vi "background writer.vi"(0 "dictionary":T2, 1 "command queue":refnum<k33>, 2 "response from processor":refnum<k33>, 5 "logging path":path, 7 "backup directory":path, 9 "default data table":T1, 11 "scans per write":u16=20, 13 "enable channel (bool)":i32, 14 "has enable channel":bool) -> (15 "error out":errorcluster)   [LabVIEW 2013, in "Binary datalogger runtime.lvclass"]
uses:
  Binary datalogger runtime.lvclass
  <vilib>/NI/Tag Bus/dictionary/full data dictionary.ctl
  message to background process.ctl
  control enum.ctl
  <vilib>/NI/Tag Bus/table/data table.ctl
  response from background process.ctl
  response enum.ctl
  writer state enum.ctl
  data cache.ctl
  <vilib>/NI/Tag Bus/table/data table.lvlib
  <vilib>/NI/Configuration Framework/serializable configuration/NISE_CEF_serializable configuration.lvclass
  <vilib>/NI/Tag Bus/dictionary/data dictionary.lvclass
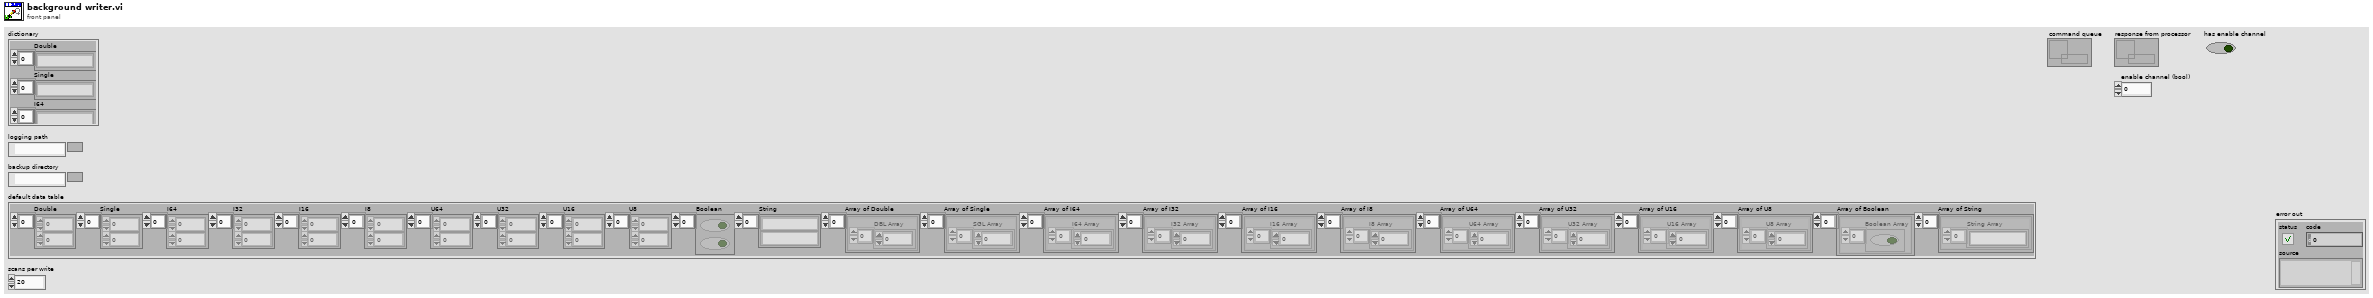
[diagram p1: front panel]
types:
  T1 = typedef "tag bus.lvlib/data table.lvlib/data table.ctl" = cluster{"Double":dbl[], "Single":sgl[], "I64":i64[], "I32":i32[], "I16":i16[], "I8":i8[], "U64":u64[], "U32":u32[], "U16":u16[], "U8":u8[], "Boolean":bool[], "String":string[], "Array of Double":cluster{"DBL Array":dbl[]}[], "Array of Single":cluster{"SGL Array":sgl[]}[], "Array of I64":cluster{"I64 Array":i64[]}[], "Array of I32":cluster{"I32 Array":i32[]}[], "Array of I16":cluster{"I16 Array":i16[]}[], "Array of I8":cluster{"I8 Array":i8[]}[], "Array of U64":cluster{"U64 Array":u64[]}[], "Array of U32":cluster{"U32 Array":u32[]}[], "Array of U16":cluster{"U16 Array":u16[]}[], "Array of U8":cluster{"U8 Array":u8[]}[], "Array of Boolean":cluster{"Boolean Array":bool[]}[], "Array of String":cluster{"String Array":string[]}[]}
  T2 = typedef "tag bus.lvlib/data dictionary.lvclass/full data dictionary.ctl" = cluster{"Double":string[], "Single":string[], "I64":string[], "I32":string[], "I16":string[], "I8":string[], "U64":string[], "U32":string[], "U16":string[], "U8":string[], "Boolean":string[], "String":string[], "Array of Double":string[], "Array of Single":string[], "Array of I64":string[], "Array of I32":string[], "Array of I16":string[], "Array of I8":string[], "Array of U64":string[], "Array of U32":string[], "Array of U16":string[], "Array of U8":string[], "Array of Boolean":string[], "Array of String":string[]}
  T3 = enum16{"open", "replace", "create", "open or create", "replace or create", "replace or create with confirmation"}
  T4 = typedef "Binary datalogger runtime.lvclass/data cache.ctl" = cluster{"timestamps":timestamp[], "dataset":T1[]}
  T5 = typedef "Binary datalogger runtime.lvclass/writer state enum.ctl" = enum16{"wait for message", "create file", "report error", "exit", "close file"}
  T6 = typedef "Binary datalogger runtime.lvclass/response enum.ctl" = enum16{"exit", "return buffer", "error"}
  T7 = typedef "Binary datalogger runtime.lvclass/response from background process.ctl" = cluster{"response enum":T6, "datapack":refnum<data-value>, "error code":i32}
  T8 = typedef "Binary datalogger runtime.lvclass/message to background process.ctl" = cluster{"control enum":T9, "datapack":refnum<data-value>, "Time Stamp":timestamp}
  T9 = typedef "Binary datalogger runtime.lvclass/control enum.ctl" = enum16{"exit", "output data"}
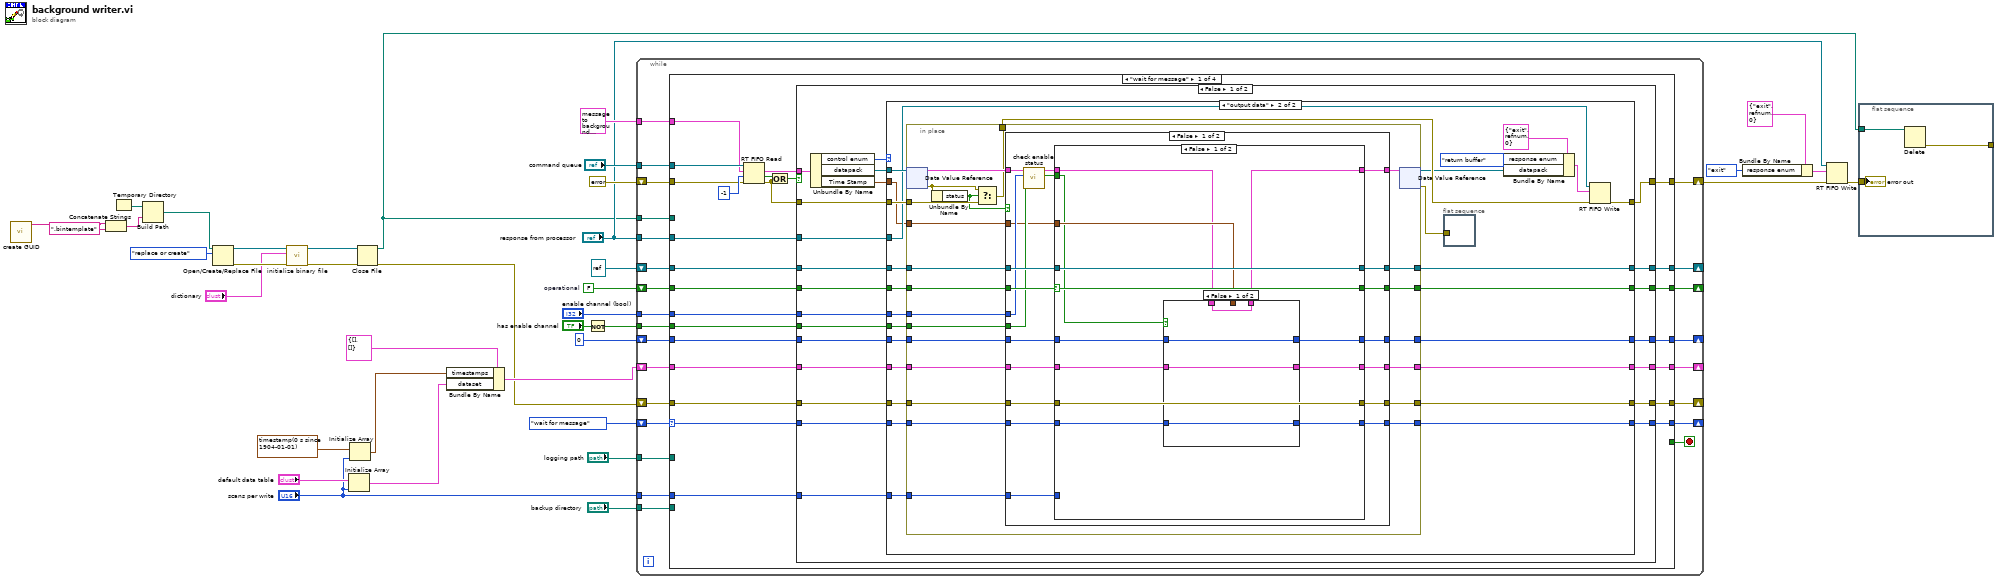
[diagram p0: block diagram]
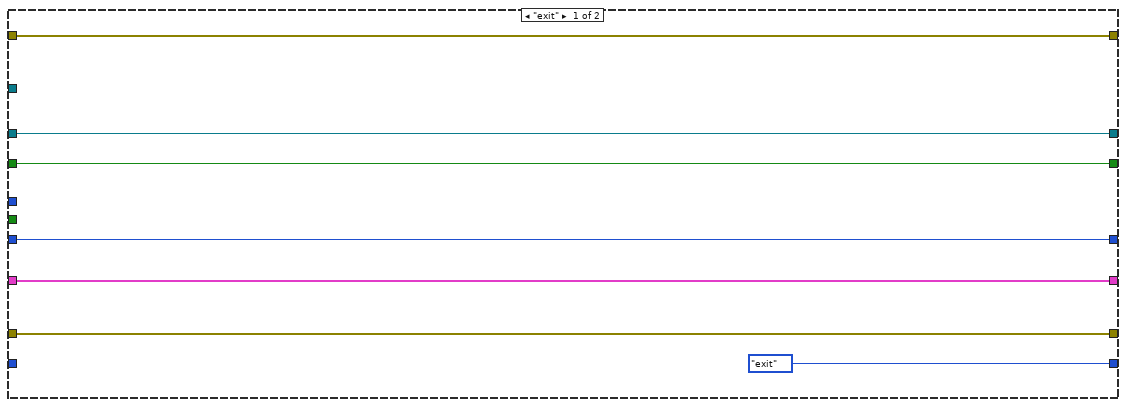
[diagram p2: hidden frame]
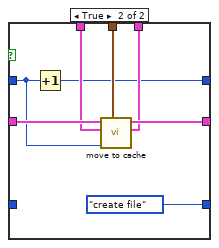
[diagram p3: hidden frame]
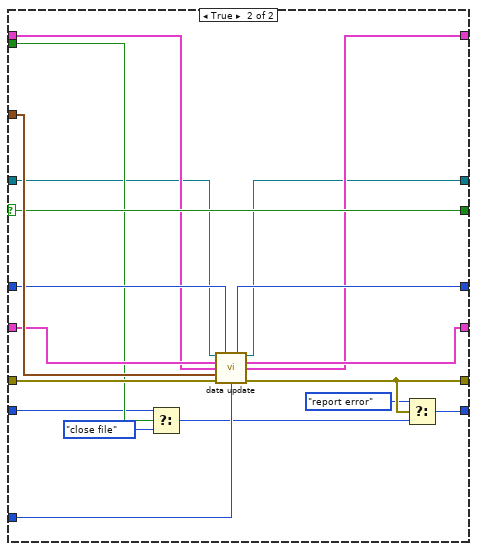
[diagram p4: hidden frame]
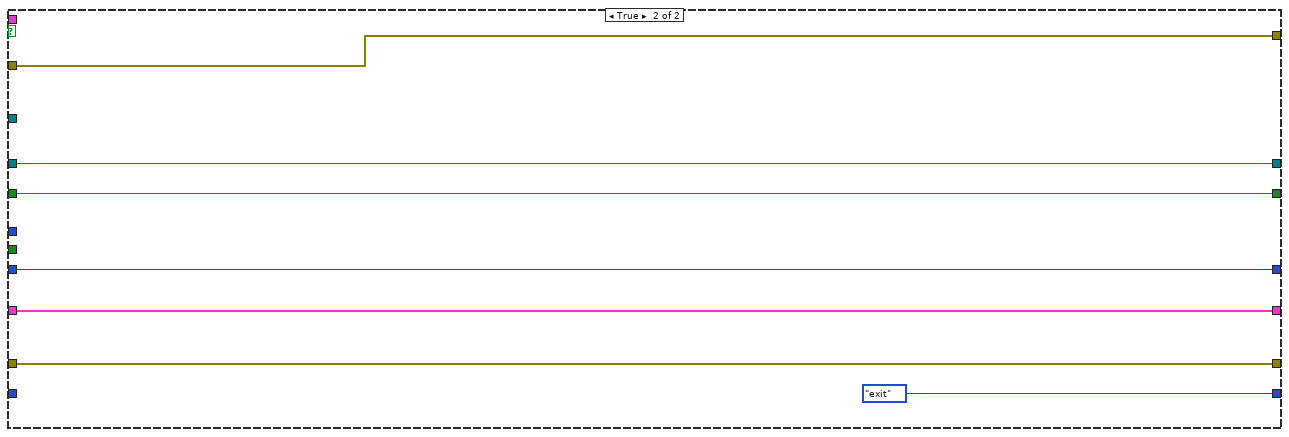
[diagram p6: hidden frame]
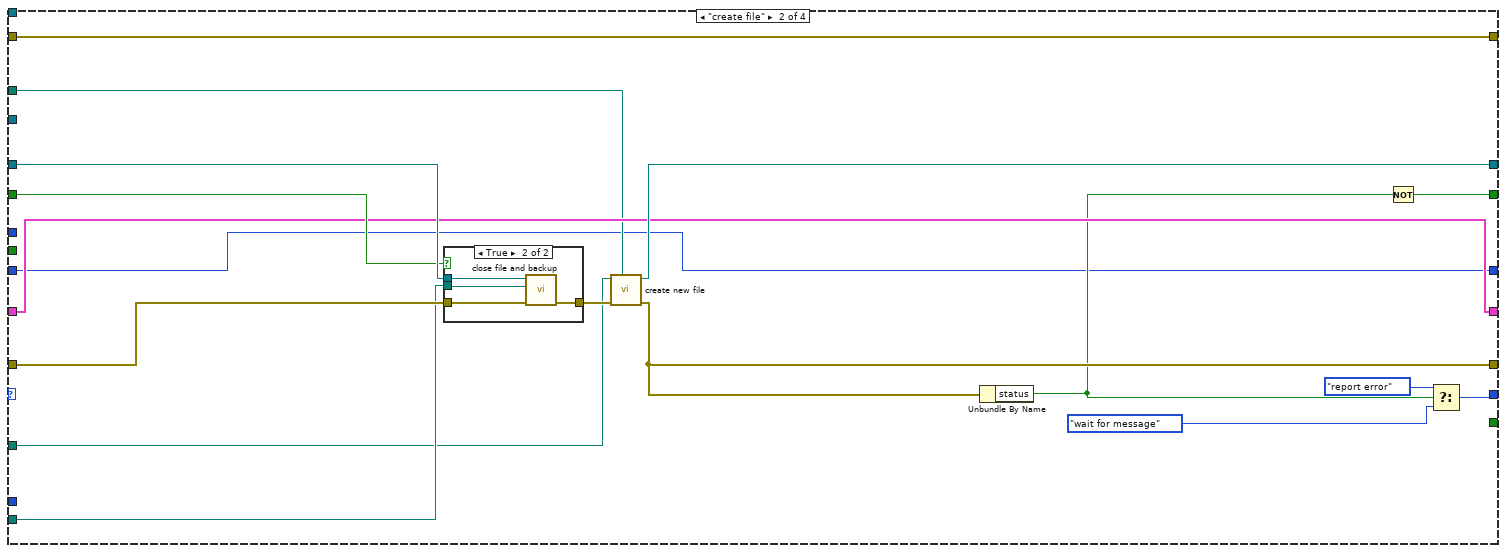
[diagram p7: hidden frame]
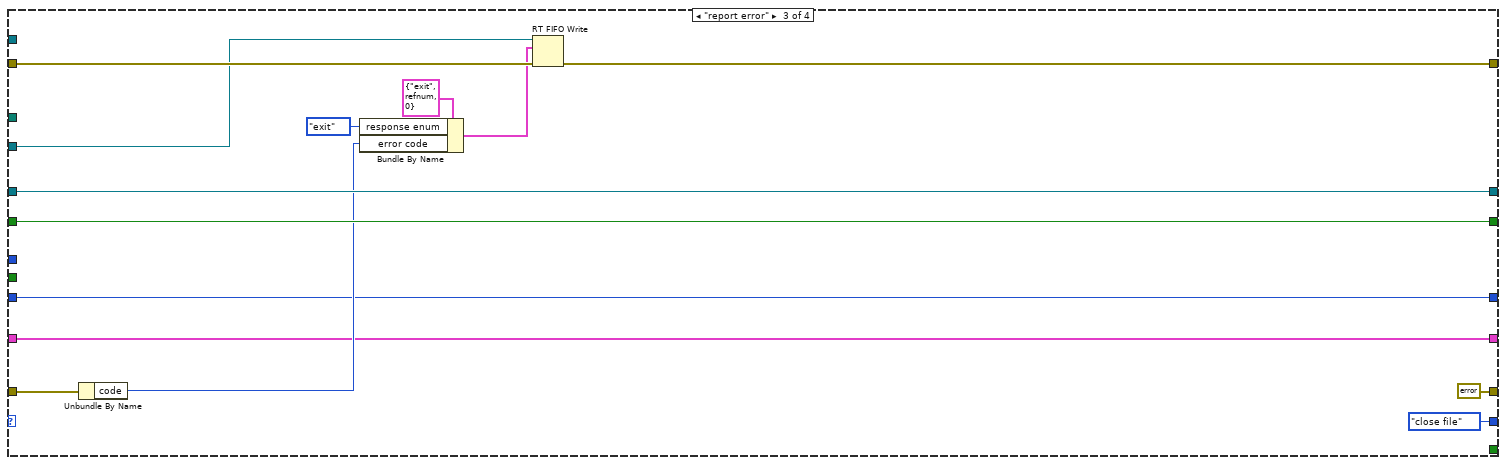
[diagram p9: hidden frame]
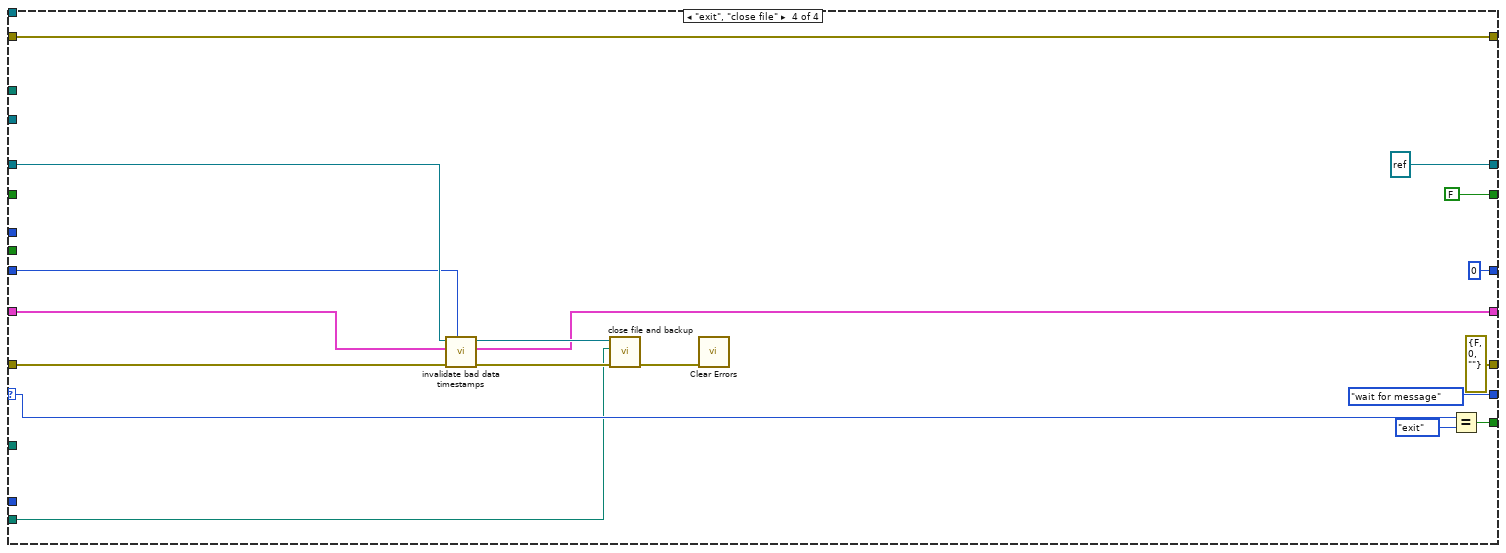
[diagram p10: hidden frame]
diagram:
  w28 = FALSE  # operational
  n1 = call <vilib>:"create GUID.vi"() -> ("uuid"=w12:string)  [unwired: 10 in, 1 out]
  n2 = Concatenate Strings(w12, ".bintemplate" ("string")) -> (w10:string)
  n3 = Temporary Directory() -> (w13:path)
  n4 = Build Path(base path=w13, name or relative path=w10) -> (appended path=w9:path)
  n5 = Open/Create/Replace File(file path (use dialog)=w9, operation (0:open)=T3."replace or create") -> (refnum out=w7:refnum<file>, error out=w6:errorcluster)  [unwired: 4 in, 1 out]
  n6 = call "initialize binary file.vi"("error in"=w6, "dictionary"="dictionary", "Byte Stream File in"=w7) -> ("error out"=w5:errorcluster, "Byte Stream File out"=w4:refnum<file>)  [unwired: 7 in]
  n7 = Initialize Array("default data table", "scans per write") -> (w17:T1[])
  n8 = Initialize Array(timestamp(0 s since 1904-01-01) ("Time Stamp"), "scans per write") -> (w14:timestamp[])
  n9 = Close File(refnum=w4, error in=w5) -> (path=w2:path, error out=w3:errorcluster)
  n10 = Bundle By Name(cluster=T4 {"timestamps"=[], "dataset"=[]} ("cache allocation in"), "timestamps"=w14, "dataset"=w17) -> (w18:T4)
  n11 = Not(x="has enable channel") -> (.not. x?=w24:bool)
  n12 = while {
    tunnel: "command queue" -> [w62]
    tunnel: T8 {"control enum"=enum."exit", "datapack"=refnum, "Time Stamp"=timestamp(0 s since 1904-01-01)} ("element") -> [w61]
    shift-right: [w59] -> w35
    shift-left: errorcluster {"status"=FALSE, "code"=0, "source"=""} ("error in") -> [w60]
    tunnel: "response from processor" -> [w57]
    shift-right: [w55] -> _
    shift-left: writer_state_enum."wait for message" ("logger state") -> [w56]
    shift-right: [w53] -> _
    shift-left: refnum<file> refnum ("refnum out") -> [w54]
    shift-right: [w46] -> _
    shift-left: w28 -> [w52]
    shift-right: [w50] -> _
    shift-left: w3 -> [w51]
    tunnel: "logging path" -> [w49]
    tunnel: "scans per write" -> [w48]
    tunnel: "backup directory" -> [w47]
    shift-right: [w45] -> _
    shift-left: 0 ("sample counter") -> [w44]
    shift-right: [w40] -> _
    shift-left: w18 -> [w41]
    tunnel: "enable channel (bool)" -> [w42]
    tunnel: w24 -> [w43]
    tunnel: w2 -> [w39]
    stop <- w58 stop-if-true
    n13 = case shown="\"wait for message\"" w56 {
      selector: w56 -> [w66 _ _ w294]
      tunnel: w62 -> [w87 _ _ _]
      tunnel: w61 -> [w85 _ _ _]
      tunnel: w60 -> [w84 w248 w278 w296]
      tunnel: [w80 w248 w276 w296] -> w59
      tunnel: [_ _ _ w295] -> w58
      tunnel: w57 -> [w78 _ w275 _]
      tunnel: [w77 w250 writer_state_enum."close file" ("logger state") writer_state_enum."wait for message" ("logger state")] -> w55
      tunnel: w54 -> [w76 w255 w277 w288]
      tunnel: [w75 w259 w277 refnum<file> refnum ("refnum out")] -> w53
      tunnel: w52 -> [w73 w247 w269 _]
      tunnel: w51 -> [w71 w256 w268 w289]
      tunnel: [w72 w258 errorcluster {"status"=FALSE, "code"=0, "source"=""} ("error out") errorcluster {"status"=FALSE, "code"=0, "source"=""} ("error out")] -> w50
      tunnel: w49 -> [_ w253 _ _]
      tunnel: w48 -> [w63 _ _ _]
      tunnel: w47 -> [_ w254 _ w287]
      tunnel: [w74 w249 w269 FALSE] -> w46
      tunnel: [w69 w243 w265 0 ("sample counter")] -> w45
      tunnel: w44 -> [w70 w243 w265 w284]
      tunnel: w43 -> [w64 _ _ _]
      tunnel: w42 -> [w65 _ _ _]
      tunnel: w41 -> [w68 w246 w266 w286]
      tunnel: [w67 w246 w266 w285] -> w40
      tunnel: w39 -> [_ w245 _ _]
      frame "wait for message" {
        n14 = RT FIFO Read(0:w87, 1:w85, 2:-1 ("timeout in ms (0)"), 3:w84) -> (9:w79:T8, 10:w83:bool, 11:w81:errorcluster)  [unwired: 2 out]
        n15 = Or(x=w83, y=w81) -> (x .or. y?=w82:bool)
        n16 = case shown="False" w82 {
          tunnel: w81 -> [w106 w242]
          tunnel: [w107 w242] -> w80
          tunnel: w79 -> [w109 _]
          tunnel: w78 -> [w103 _]
          tunnel: [w102 writer_state_enum."exit" ("logger state")] -> w77
          tunnel: w76 -> [w101 w240]
          tunnel: [w100 w240] -> w75
          tunnel: [w98 w239] -> w74
          tunnel: w73 -> [w99 w239]
          tunnel: [w97 w238] -> w72
          tunnel: w71 -> [w96 w238]
          tunnel: w70 -> [w94 w237]
          tunnel: [w95 w237] -> w69
          tunnel: w68 -> [w93 w236]
          tunnel: [w92 w236] -> w67
          tunnel: w66 -> [w91 _]
          tunnel: w65 -> [w90 _]
          tunnel: w64 -> [w89 _]
          tunnel: w63 -> [w88 _]
          frame False {
            n17 = Unbundle By Name(w109) -> ("control enum"=w108:T9, "datapack"=w104:refnum<data-value>, "Time Stamp"=w105:timestamp)
            n18 = case shown="\"output data\"" w108 {
              tunnel: [w116 w126] -> w107
              tunnel: w106 -> [w116 w141]
              tunnel: w105 -> [_ w118]
              tunnel: w104 -> [_ w142]
              tunnel: w103 -> [_ w123]
              tunnel: [writer_state_enum."exit" ("logger state") w130] -> w102
              tunnel: w101 -> [w114 w140]
              tunnel: [w114 w139] -> w100
              tunnel: w99 -> [w113 w137]
              tunnel: [w113 w138] -> w98
              tunnel: [w112 w131] -> w97
              tunnel: w96 -> [w112 w132]
              tunnel: [w110 w135] -> w95
              tunnel: w94 -> [w110 w136]
              tunnel: w93 -> [w111 w133]
              tunnel: [w111 w134] -> w92
              tunnel: w91 -> [_ w129]
              tunnel: w90 -> [_ w128]
              tunnel: w89 -> [_ w127]
              tunnel: w88 -> [_ w117]
              frame "exit" {
              }
              frame "output data" {
                n19 = in-place {
                  in-place-border: w141 -> [w164]
                  in-place-border: w140 -> [w159]
                  in-place-border: [w158] -> w139
                  in-place-border: [w157] -> w138
                  in-place-border: w137 -> [w156]
                  in-place-border: w136 -> [w155]
                  in-place-border: [w154] -> w135
                  in-place-border: [w153] -> w134
                  in-place-border: w133 -> [w152]
                  in-place-border: w132 -> [w151]
                  in-place-border: [w150] -> w131
                  in-place-border: [w149] -> w130
                  in-place-border: w129 -> [w148]
                  in-place-border: [w147] -> w125
                  in-place-border: w128 -> [w146]
                  in-place-border: w127 -> [w145]
                  in-place-border: w118 -> [w144]
                  in-place-border: w117 -> [w143]
                  n20 = in-place-dvr #1(w142) -> (w160:T1, w163:errorcluster)
                  n21 = Unbundle By Name(w163) -> ("status"=w162:bool)
                  n22 = Select(t=w163, s=w162, f=w164) -> (s? t:f=w147:errorcluster)
                  n23 = case shown="False" w162 {
                    tunnel: [w169 w235] -> w161
                    tunnel: w160 -> [w172 w235]
                    tunnel: w159 -> [w181 w234]
                    tunnel: [w182 w234] -> w158
                    tunnel: [w183 w233] -> w157
                    tunnel: w156 -> [w184 w233]
                    tunnel: w155 -> [w179 w232]
                    tunnel: [w180 w232] -> w154
                    tunnel: [w175 w231] -> w153
                    tunnel: w152 -> [w176 w231]
                    tunnel: w151 -> [w178 w230]
                    tunnel: [w177 w230] -> w150
                    tunnel: [w174 w229] -> w149
                    tunnel: w148 -> [w173 w229]
                    tunnel: w146 -> [w168 _]
                    tunnel: w145 -> [w167 _]
                    tunnel: w144 -> [w166 _]
                    tunnel: w143 -> [w165 _]
                    frame False {
                      n24 = call "check enable status.vi"("always enabled?"=w167, "enable channel index"=w168, "data table in"=w172) -> ("enabled?"=w170:bool, "Data table out"=w171:T1)  [unwired: 7 in]
                      n25 = case shown="False" w184 {
                        selector: w184 -> [w197 w222]
                        tunnel: [w197 w222] -> w183
                        tunnel: [w196 w210] -> w182
                        tunnel: w181 -> [w196 w211]
                        tunnel: [w188 w224] -> w180
                        tunnel: w179 -> [w187 w225]
                        tunnel: w178 -> [w195 w228]
                        tunnel: [w195 w221] -> w177
                        tunnel: w176 -> [w193 w226]
                        tunnel: [w192 w223] -> w175
                        tunnel: [w186 w220] -> w174
                        tunnel: w173 -> [w185 w214]
                        tunnel: w171 -> [w191 w217]
                        tunnel: w170 -> [w189 w215]
                        tunnel: [w190 w218] -> w169
                        tunnel: w166 -> [w194 w227]
                        tunnel: w165 -> [_ w216]
                        frame False {
                          n26 = case shown="False" w189 {
                            tunnel: w194 -> [_ w209]
                            tunnel: w193 -> [w200 w208]
                            tunnel: [w200 w207] -> w192
                            tunnel: w191 -> [w201 w206]
                            tunnel: [w201 w205] -> w190
                            tunnel: [w198 w203] -> w188
                            tunnel: w187 -> [w198 w202]
                            tunnel: [w199 writer_state_enum."create file" ("logger state")] -> w186
                            tunnel: w185 -> [w199 _]
                            frame False {
                            }
                            frame True {
                              n27 = Increment(x=w202) -> (x+1=w203:i32)
                              n28 = call "move to cache.vi"("Time Stamp"=w209, "sample counter"=w202, "data table in"=w206, "cache in"=w208) -> ("data table out"=w205:T1, "cache out"=w207:T4)  [unwired: 6 in]
                            }
                          }
                        }
                        frame True {
                          n29 = Select(t=w214, s=w215, f=writer_state_enum."close file") -> (s? t:f=w212:T5)
                          n30 = call "data update.vi"("bin in"=w211, "sample counter in"=w225, "cache in"=w226, "data table in"=w217, "Time Stamp"=w227, "error in"=w228, "scans per write"=w216) -> ("sample counter out"=w224:i32, "bin out"=w210:refnum<file>, "cache out"=w223:T4, "data table out"=w218:T1, "error out"=w221:errorcluster)  [unwired: 4 in]
                          n31 = Select(t=writer_state_enum."report error", s=w221, f=w212) -> (s? t:f=w220:T5)
                        }
                      }
                    }
                    frame True {
                    }
                  }
                  n32 = in-place-dvr #1(w161) -> (w120:refnum<data-value>, w124:errorcluster)
                }
                n33 = flat-sequence {
                  tunnel: w124 -> [_]
                  frame #0 {
                  }
                }
                n34 = Bundle By Name(cluster=T7 {"response enum"=enum."exit", "datapack"=refnum, "error code"=0} ("element"), "response enum"=response_enum."return buffer", "datapack"=w120) -> (w121:T7)
                n35 = RT FIFO Write(0:w123, 1:w121, 3:w125) -> (11:w126:errorcluster)  [unwired: 2 in, 3 out]
              }
            }
          }
          frame True {
          }
        }
      }
      frame "create file" {
        n36 = case shown="True" w247 {
          tunnel: [w260 w263] -> w257
          tunnel: w256 -> [w260 w264]
          tunnel: w255 -> [_ w262]
          tunnel: w254 -> [_ w261]
          frame False {
          }
          frame True {
            n37 = call "close file and backup.vi"("error in"=w264, "backup directory"=w261, "bin file in"=w262) -> ("error out"=w263:errorcluster)  [unwired: 8 in]
          }
        }
        n38 = call "create new file.vi"("template path"=w245, "error in"=w257, "logging path"=w253) -> ("error out"=w258:errorcluster, "bin file out"=w259:refnum<file>)  [unwired: 7 in]
        n39 = Unbundle By Name(w258) -> ("status"=w244:bool)
        n40 = Not(x=w244) -> (.not. x?=w249:bool)
        n41 = Select(t=writer_state_enum."report error" ("logger state"), s=w244, f=writer_state_enum."wait for message" ("logger state")) -> (s? t:f=w250:T5)
      }
      frame "report error" {
        n42 = Unbundle By Name(w268) -> ("code"=w267:i32)
        n43 = Bundle By Name(cluster=T7 {"response enum"=enum."exit", "datapack"=refnum, "error code"=0} ("element"), "response enum"=response_enum."exit", "error code"=w267) -> (w273:T7)
        n44 = RT FIFO Write(0:w275, 1:w273, 3:w278) -> (11:w276:errorcluster)  [unwired: 2 in, 3 out]
      }
      frame "exit", "close file" {
        n45 = call "invalidate bad data timestamps.vi"("sample counter"=w284, "error in"=w289, "cache allocation in"=w286, "bin file in"=w288) -> ("error out"=w290:errorcluster, "cache allocation out"=w285:T4, "bin file out"=w291:refnum<file>)  [unwired: 5 in]
        n46 = call "close file and backup.vi"("error in"=w290, "backup directory"=w287, "bin file in"=w291) -> ("error out"=w281:errorcluster)  [unwired: 8 in]
        n47 = call <vilib>:"Clear Errors.vi"("error in (no error)"=w281) -> ()  [unwired: 6 in, 1 out]
        n48 = Equal?(x=w294, y=writer_state_enum."exit") -> (x = y?=w295:bool)
      }
    }
  }
  n49 = Bundle By Name(cluster=T7 {"response enum"=enum."exit", "datapack"=refnum, "error code"=0} ("element"), "response enum"=response_enum."exit") -> (w32:T7)
  n50 = RT FIFO Write(0:"response from processor", 1:w32, 3:w35) -> (11:w30:errorcluster)  [unwired: 2 in, 3 out]
  n51 = flat-sequence {
    tunnel: w30 -> [w299]
    tunnel: w2 -> [w298]
    tunnel: [w297] -> _
    frame #0 {
      n52 = Delete(path (use dialog)=w298) -> (error out=w297:errorcluster)  [unwired: 4 in, 2 out]
      "error out" <- w299
    }
  }
